vi "Backprop_grads.vi"(0 "Activation":T1, 1 "m":dbl format="%#_13g", 2 "dA_l":T2, 3 "W_l":T2, 4 "A_l-1":T2, 5 "A_l":T2) -> (6 "dA_l-1":T2, 7 "dW_l":T2, 8 "db_l":T2)   [LabVIEW 2016]
uses:
  <vilib>/Analysis/Matrix/Datatypes/RealMatrix.ctl
  Enum_activations.ctl
  <vilib>/Analysis/Matrix/NI_Matrix.lvlib
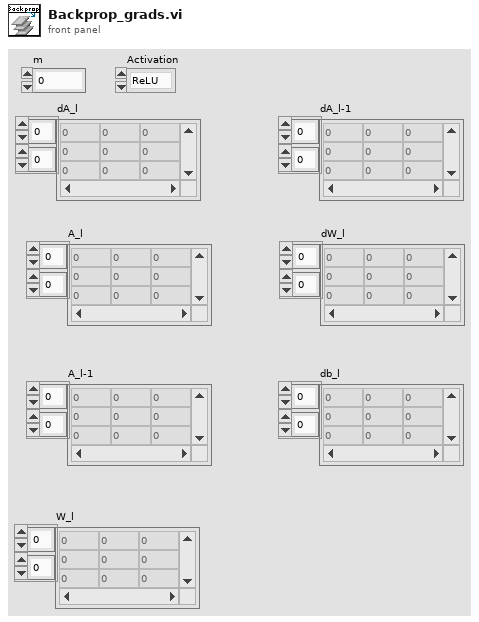
[diagram p1: front panel]
types:
  T1 = typedef "Enum_activations.ctl" = enum16{"ReLU", "Sigmoid"}
  T2 = typedef "NI_Matrix.lvlib/RealMatrix.ctl" = dbl[][]
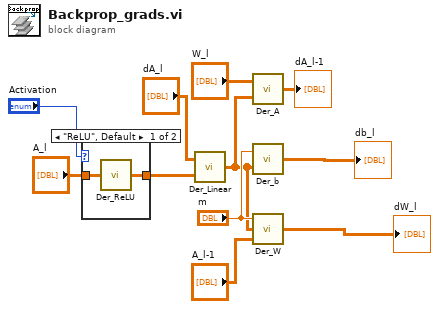
[diagram p0: block diagram]
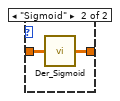
[diagram p2: hidden frame]
diagram:
  n1 = case shown="\"ReLU\", Default" "Activation" {
    tunnel: "A_l" -> [w13 w15]
    tunnel: [w12 w14] -> w8
    frame "ReLU", Default {
      n2 = call "Der_ReLU.vi"("A_l"=w13) -> ("g'(Z)"=w12:T2)
    }
    frame "Sigmoid" {
      n3 = call "Der_Sigmoid.vi"("A_l"=w15) -> ("g'(Z)"=w14:T2)
    }
  }
  n4 = call "Der_Linear.vi"("g'(z)"=w8, "dA_l"="dA_l") -> ("dZ_l"=w1:T2)
  n5 = call "Der_A.vi"("dZ_l"=w1, "W_l"="W_l") -> ("dA_l-1"=→"dA_l-1":T2)
  n6 = call "Der_b.vi"("dZ_l"=w1, "m"="m") -> ("db_l"=→"db_l":T2)
  n7 = call "Der_W.vi"("dA_l-1"="A_l-1", "dZ_l"=w1, "m"="m") -> ("dW_l"=→"dW_l":T2)
